vi "AO Python Get Image.vi"(0 "Camera Notifier":string) -> (8 "Image Out":dbl[][][](array[numeric]))   [LabVIEW 2016]
uses:
  Device Library/Cameras/Hamamatsu/Orca Flash/Orca Flash Controls/Orca Flash Actions.ctl
  Device Library/Cameras/Camera Controls/Camera IMAQ Key Info.ctl
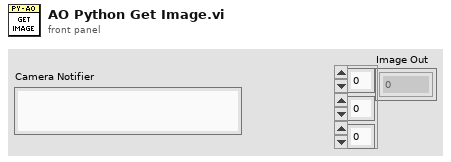
[diagram p1: front panel]
types:
  T1 = typedef "Image Type" = u32
  T2 = typedef "Camera IMAQ Key Info.ctl" = cluster{"Frame":u32, "Sensor Height":i32, "Sensor Width":i32, "ROI Height":i32, "ROI Width":i32, "ROI Enable?":bool, "Bit per Pixel":u8}
  T3 = typedef "Orca Flash Actions.ctl" = enum16{"IDLE", "PREVIEW", "RECORD", "Record Settings", "SETPARAM", "GETPARAM", "SETROI", "GETROI", "PROGRESSIVE MODE", "AREA MODE", "STATUS", "QUIT"}
  T4 = typedef "IMAQ Image.ctl" = refnum<image>
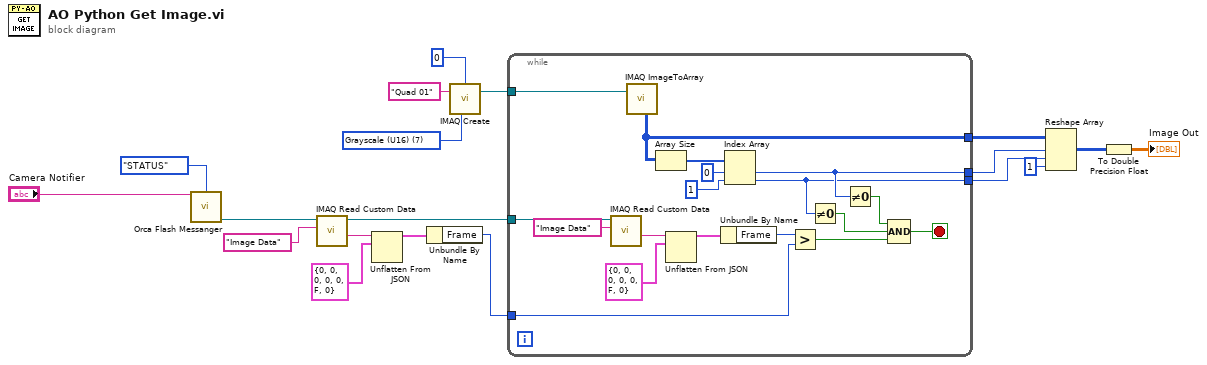
[diagram p0: block diagram]
diagram:
  w2 = T1 7 items=["Grayscale (U8)", "Grayscale (I16)", "Grayscale (SGL)", "Complex (CSG)", "RGB (U32)", "HSL (U32)", "RGB (U64)", "Grayscale (U16)"] ("Image Type")
  n1 = call "Orca Flash Messanger.vi"("Notifier Name"="Camera Notifier", "Camera Actions"=Orca_Flash_Actions."STATUS") -> ("Image Ref"=w17:T4)  [unwired: 9 in, 4 out]
  n2 = call "IMAQ Read Custom Data"("Key"="Image Data", "Image"=w17) -> ("Custom Data Out"=w15:string, "Image (duplicate)"=w12:T4)  [unwired: 7 in, 1 out]
  n3 = Unflatten From JSON(JSON string=w15, type and defaults=T2 {"Frame"=0, "Sensor Height"=0, "Sensor Width"=0, "ROI Height"=0, "ROI Width"=0, "ROI Enable?"=FALSE, "Bit per Pixel"=0} ("Camera IMAQ Key Info")) -> (value=w13:T2)  [unwired: 5 in, 1 out]
  n4 = Unbundle By Name(w13) -> ("Frame"=w11:u32)
  n5 = call "IMAQ Create"("Border Size"=0, "Image Name"="Quad 01", "Image Type"=w2) -> ("New Image"=w1:T4)  [unwired: 2 in, 1 out]
  n6 = while {
    tunnel: w12 -> [w33]
    tunnel: w11 -> [w31]
    tunnel: [w27] -> w8
    tunnel: [w24] -> w6
    tunnel: [w22] -> w7
    tunnel: w1 -> [w20]
    stop <- w25 stop-if-true
    n7 = call "IMAQ Read Custom Data"("Key"="Image Data", "Image"=w33) -> ("Custom Data Out"=w36:string)  [unwired: 7 in, 2 out]
    n8 = call "IMAQ ImageToArray"("Image"=w20) -> ("Image Pixels (U16)"=w27:u16[][])  [unwired: 3 in, 4 out]
    n9 = Array Size(array=w27) -> (size(s)=w30:i32[])
    n10 = Unflatten From JSON(JSON string=w36, type and defaults=T2 {"Frame"=0, "Sensor Height"=0, "Sensor Width"=0, "ROI Height"=0, "ROI Width"=0, "ROI Enable?"=FALSE, "Bit per Pixel"=0} ("Camera IMAQ Key Info")) -> (value=w34:T2)  [unwired: 5 in, 1 out]
    n11 = Unbundle By Name(w34) -> ("Frame"=w32:u32)
    n12 = Index Array(array=w30, index #1=0 ("index"), index #2=1 ("index")) -> (element #1=w24:i32, element #2=w22:i32)
    n13 = Greater?(x=w32, y=w31) -> (0:w26:bool)
    n14 = Not Equal To 0?(x=w22) -> (x != 0?=w21:bool)
    n15 = Not Equal To 0?(x=w24) -> (x != 0?=w23:bool)
    n16 = Compound Arithmetic op=AND(w23, w21, w26) -> (w25:bool)
  }
  n17 = Reshape Array(w8, w6, w7, 1 ("dimension size")) -> (w5:u16[][][])
  n18 = To Double Precision Float(number=w5) -> (double precision float=→"Image Out":dbl[][][])
